vi "EOL All-Station All-Channel Buffer.vi"(9 "station idx":i32=4, 10 "Data Index In":i32, 11 "All Data In":dbl[][](array[numeric])) -> (2 "Data Index Out":i32, 3 "All Data Out":dbl[][](array[numeric]))   [LabVIEW 2012]
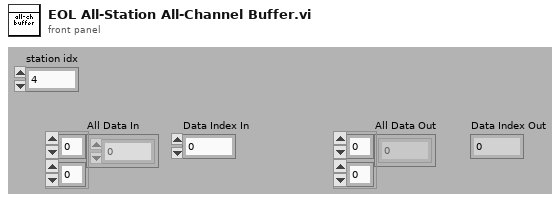
[diagram p1: front panel]
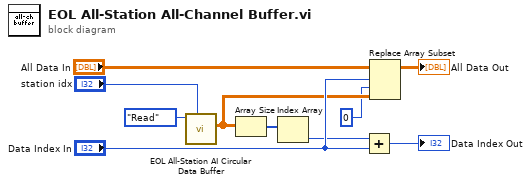
[diagram p0: block diagram]
diagram:
  n1 = call "EOL All-Station AI Circular Data Buffer.vi"("station idx"="station idx", "Mode"=enum16{"Initialize", "Read", "Write"}."Read") -> ("Data Read (Samp-Ro, Ch-Col)"=w2:dbl[][])  [unwired: 9 in]
  n2 = Array Size(array=w2) -> (size(s)=w4:i32[])
  n3 = Index Array(array=w4) -> (element=w3:i32)  [unwired: 1 in]
  n4 = Add(x=w3, y="Data Index In") -> (x+y=→"Data Index Out":i32)
  n5 = Replace Array Subset(array="All Data In", new element=w2, index (row)="Data Index In", index (col)=0 ("disabled index (col)")) -> (→"All Data Out":dbl[][])
